vi "Bildaufnahme_Oben.vi"(8 "Fehler in":errorcluster, 11 "Cluster in":T1={"Initialisierung"={"Online?"=FALSE, "Grundpfad"=path "", "Kamera Oben"="", "IP-Adresse Flüssiglinse"="", "Flüssiglinse"=refnum, "Kamera Unten"="", "IP-Adresse SPS"="", "SPS-Verbindung"={"TCP Connection Ref"=refnum, "IP address"="", "timeout ms"=5000, "Connected?"=FALSE, "PLC Type"=enum."S7 1200", "Rack S7 400"=0, "Slot S7 400"=0, "PDU Size"=0, "connection semaphore"=refnum}, "IP-Adresse Lichtgitter"="", "Lichtgitter"=refnum, "Skalierungsfaktor"=0.0, "Bilder Oben"=[], "Bild Unten"=refnum, "Bild Ausschnitt Unten"=refnum}, "Einstellungen"={"Gesamtablauf gestartet"=FALSE, "i. O. Bilder speichern"=FALSE, "Bildspeicherung Offline"=FALSE, "Ausgewähltes Offline-Datum"="", "Ausgewähltes Offline-Teil"="", "Speicherpfad Bilder"=path ""}, "Artikeldaten"={"Artikelnummer"="", "Fertigungsauftrag"="", "Muster ISO"=refnum, "Belichtungszeit Referenzmarken"=0.0, "Fokus Referenzmarken"=0.0, "Belichtungszeit ISO"=0.0, "Fokus ISO"=0.0, "Belichtungszeit Unten"=0.0, "Kontaktanzahl"=0, "Aktueller Kontakt"=0, "Kontaktposition"={"x"=0.0, "y"=0.0}, "ISO-Muster nicht vorhanden"=FALSE, "Winkel ISO"=0.0, "Mittelpunkt ISO"={"x"=0.0, "y"=0.0}}, "Werte Kamera Oben"={"Koordinatensystem"={"Punkt x-Achse"={"X"=0.0, "Y"=0.0}, "Ursprung"={"X"=0.0, "Y"=0.0}, "Punkt y-Achse"={"X"=0.0, "Y"=0.0}}, "Position Kontakt"={"x"=0.0, "y"=0.0}, "Durchmesser Loch"=0.0, "Winkel Kontakt"=0.0, "Position Kontakt umgerechnet"={"x"=0.0, "y"=0.0}}, "Werte Kamera Unten"={"Prüfung Unten n. i. O."=FALSE}, "Werte Lichtgitter"={"Messwerte Referenzmarken"=[], "Mittelpunkt Referenzmarken"={"x"=0.0, "y"=0.0}, "Messwerte Kontakt"=[], "Offset"={"x"=0.0, "y"=0.0}}, "Rückmeldungen"={"Koordinaten ermittelt"=FALSE, "Vermessung Lichtgitter fertig"=FALSE, "Nachkontrolle Kamera Unten fertig"=FALSE}, "Fehler"={"Referenzen nicht gefunden"=FALSE, "Kontakt nicht gefunden"=FALSE, "Referenzen nicht in Lichtgitter"=FALSE, "Kontakt zu groß"=FALSE, "Kontakt zu klein"=FALSE}, "Statistik"={"Statistiken"=[]}, "Timer"={"Timer Start Position"=0, "Timer Start Lichtgitter"=0, "Timer Start Kamera Unten"=0}}) -> (0 "Fehler out":errorcluster, 3 "Cluster out":T1={"Initialisierung"={"Online?"=FALSE, "Grundpfad"=path "", "Kamera Oben"="", "IP-Adresse Flüssiglinse"="", "Flüssiglinse"=refnum, "Kamera Unten"="", "IP-Adresse SPS"="", "SPS-Verbindung"={"TCP Connection Ref"=refnum, "IP address"="", "timeout ms"=5000, "Connected?"=FALSE, "PLC Type"=enum."S7 1200", "Rack S7 400"=0, "Slot S7 400"=0, "PDU Size"=0, "connection semaphore"=refnum}, "IP-Adresse Lichtgitter"="", "Lichtgitter"=refnum, "Skalierungsfaktor"=0.0, "Bilder Oben"=[], "Bild Unten"=refnum, "Bild Ausschnitt Unten"=refnum}, "Einstellungen"={"Gesamtablauf gestartet"=FALSE, "i. O. Bilder speichern"=FALSE, "Bildspeicherung Offline"=FALSE, "Ausgewähltes Offline-Datum"="", "Ausgewähltes Offline-Teil"="", "Speicherpfad Bilder"=path ""}, "Artikeldaten"={"Artikelnummer"="", "Fertigungsauftrag"="", "Muster ISO"=refnum, "Belichtungszeit Referenzmarken"=0.0, "Fokus Referenzmarken"=0.0, "Belichtungszeit ISO"=0.0, "Fokus ISO"=0.0, "Belichtungszeit Unten"=0.0, "Kontaktanzahl"=0, "Aktueller Kontakt"=0, "Kontaktposition"={"x"=0.0, "y"=0.0}, "ISO-Muster nicht vorhanden"=FALSE, "Winkel ISO"=0.0, "Mittelpunkt ISO"={"x"=0.0, "y"=0.0}}, "Werte Kamera Oben"={"Koordinatensystem"={"Punkt x-Achse"={"X"=0.0, "Y"=0.0}, "Ursprung"={"X"=0.0, "Y"=0.0}, "Punkt y-Achse"={"X"=0.0, "Y"=0.0}}, "Position Kontakt"={"x"=0.0, "y"=0.0}, "Durchmesser Loch"=0.0, "Winkel Kontakt"=0.0, "Position Kontakt umgerechnet"={"x"=0.0, "y"=0.0}}, "Werte Kamera Unten"={"Prüfung Unten n. i. O."=FALSE}, "Werte Lichtgitter"={"Messwerte Referenzmarken"=[], "Mittelpunkt Referenzmarken"={"x"=0.0, "y"=0.0}, "Messwerte Kontakt"=[], "Offset"={"x"=0.0, "y"=0.0}}, "Rückmeldungen"={"Koordinaten ermittelt"=FALSE, "Vermessung Lichtgitter fertig"=FALSE, "Nachkontrolle Kamera Unten fertig"=FALSE}, "Fehler"={"Referenzen nicht gefunden"=FALSE, "Kontakt nicht gefunden"=FALSE, "Referenzen nicht in Lichtgitter"=FALSE, "Kontakt zu groß"=FALSE, "Kontakt zu klein"=FALSE}, "Statistik"={"Statistiken"=[]}, "Timer"={"Timer Start Position"=0, "Timer Start Lichtgitter"=0, "Timer Start Kamera Unten"=0}})   [LabVIEW 2024]
doc: "Nimmt die Bilder für die Prüfung Oben auf, bzw. lädt die Bilder aus den Dateien wenn im \"Offline-Modus\"."
uses:
  Typdefinitionen/Cluster.ctl
  <vilib>/userDefined/High Color/IMAQdx.ctl
  <vilib>/DATA AHEAD/SP7/typedefs/S7 Connection.ctl
  <vilib>/DATA AHEAD/SP7/typedefs/PLC Type.ctl
  <vilib>/vision/Image Controls.llb/IMAQ Image.ctl
  Typdefinitionen/Koordinatensystem.ctl
  Typdefinitionen/Statistik.ctl
  <vilib>/vision/driver/IMAQdx.llb/IMAQdx Buffer Number Mode.ctl
  <resource>/objmgr/imaqdx.rc
  <vilib>/vision/driver/NI_Vision_Acquisition_Software.lvlib
  <vilib>/vision/NI_Vision_Development_Module.lvlib
  <vilib>/DATA AHEAD/SP7/SP7.lvlib
panel:
  in  "Zeit für Fokus":u32=300
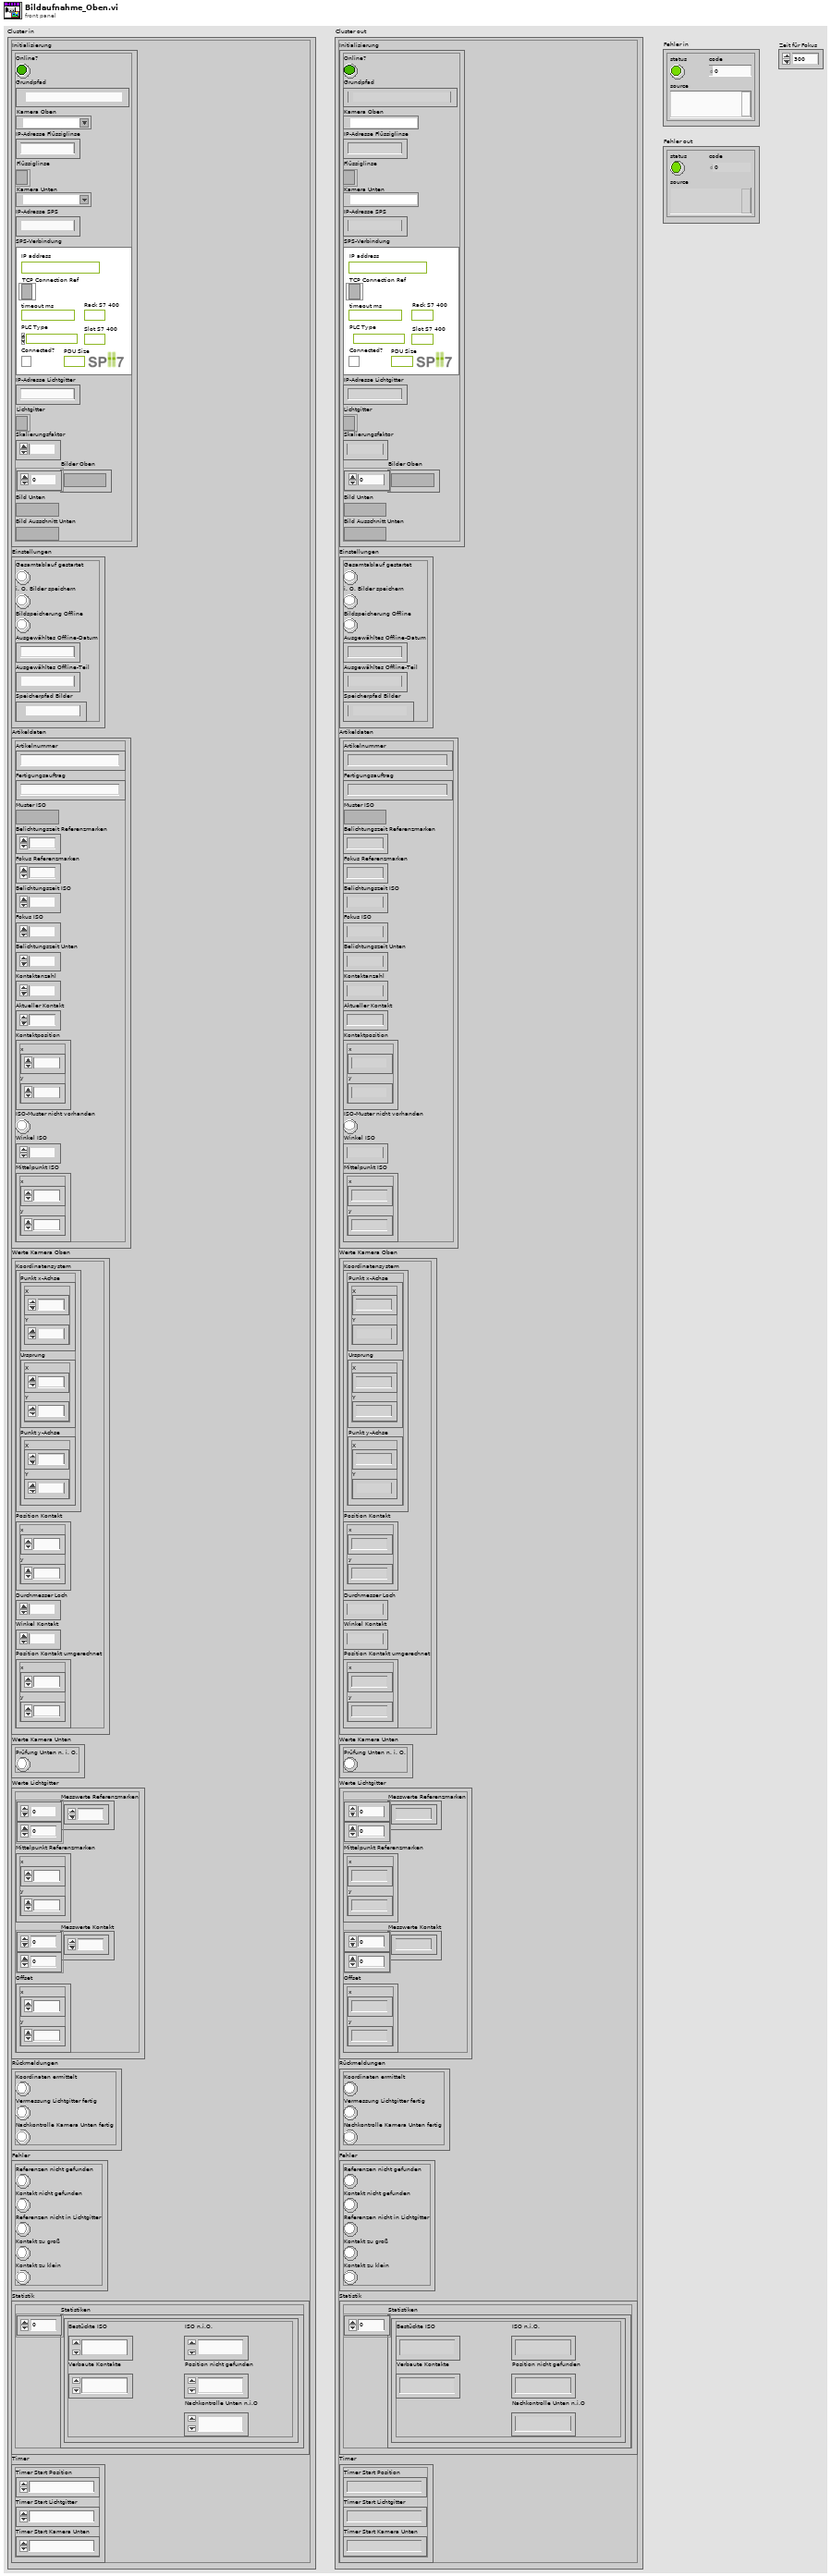
[diagram p1: front panel]
types:
  T1 = typedef "Cluster.ctl" = cluster{"Initialisierung":cluster{"Online?":bool, "Grundpfad":path, "Kamera Oben":T2, "IP-Adresse Flüssiglinse":string, "Flüssiglinse":refnum<k5>, "Kamera Unten":T2, "IP-Adresse SPS":string, "SPS-Verbindung":T3, "IP-Adresse Lichtgitter":string, "Lichtgitter":refnum<k5>, "Skalierungsfaktor":dbl, "Bilder Oben":T6[], "Bild Unten":T6, "Bild Ausschnitt Unten":T6}, "Einstellungen":cluster{"Gesamtablauf gestartet":bool, "i. O. Bilder speichern":bool, "Bildspeicherung Offline":bool, "Ausgewähltes Offline-Datum":string, "Ausgewähltes Offline-Teil":string, "Speicherpfad Bilder":path}, "Artikeldaten":cluster{"Artikelnummer":string, "Fertigungsauftrag":string, "Muster ISO":T6, "Belichtungszeit Referenzmarken":dbl, "Fokus Referenzmarken":dbl, "Belichtungszeit ISO":dbl, "Fokus ISO":dbl, "Belichtungszeit Unten":dbl, "Kontaktanzahl":u32, "Aktueller Kontakt":i16, "Kontaktposition":cluster{"x":sgl, "y":sgl}, "ISO-Muster nicht vorhanden":bool, "Winkel ISO":sgl, "Mittelpunkt ISO":cluster{"x":dbl, "y":dbl}}, "Werte Kamera Oben":cluster{"Koordinatensystem":T7, "Position Kontakt":cluster{"x":dbl, "y":dbl}, "Durchmesser Loch":dbl, "Winkel Kontakt":dbl, "Position Kontakt umgerechnet":cluster{"x":dbl, "y":dbl}}, "Werte Kamera Unten":cluster{"Prüfung Unten n. i. O.":bool}, "Werte Lichtgitter":cluster{"Messwerte Referenzmarken":dbl[][], "Mittelpunkt Referenzmarken":cluster{"x":dbl, "y":dbl}, "Messwerte Kontakt":dbl[][], "Offset":cluster{"x":dbl, "y":dbl}}, "Rückmeldungen":cluster{"Koordinaten ermittelt":bool, "Vermessung Lichtgitter fertig":bool, "Nachkontrolle Kamera Unten fertig":bool}, "Fehler":cluster{"Referenzen nicht gefunden":bool, "Kontakt nicht gefunden":bool, "Referenzen nicht in Lichtgitter":bool, "Kontakt zu groß":bool, "Kontakt zu klein":bool}, "Statistik":cluster{"Statistiken":T8[]}, "Timer":cluster{"Timer Start Position":u32, "Timer Start Lichtgitter":u32, "Timer Start Kamera Unten":u32}}
  T2 = typedef "IMAQdx.ctl" = refnum<k21>
  T3 = typedef "SP7.lvlib/S7 Connection.ctl" = cluster{"TCP Connection Ref":refnum<k5>, "IP address":string, "timeout ms":i32, "Connected?":bool, "PLC Type":T4, "Rack S7 400":u8, "Slot S7 400":u8, "PDU Size":u16, "connection semaphore":T5}
  T4 = typedef "SP7.lvlib/PLC Type.ctl" = enum16{"S7 200", "S7 300/400", "S7 1200", "S7 1500", "LOGO!8"}
  T5 = typedef "Semaphore RefNum" = refnum<k1>
  T6 = typedef "IMAQ Image.ctl" = refnum<image>
  T7 = typedef "Koordinatensystem.ctl" = cluster{"Punkt x-Achse":cluster{"X":sgl, "Y":sgl}, "Ursprung":cluster{"X":sgl, "Y":sgl}, "Punkt y-Achse":cluster{"X":sgl, "Y":sgl}}
  T8 = typedef "Statistik.ctl" = cluster{"Bestückte ISO":u32, "Verbaute Kontakte":u32, "ISO n.i.O.":u32, "Nachkontrolle Unten n.i.O":u32, "Position nicht gefunden":u32}
  T9 = typedef "IMAQ Rectangle" = cluster{"Left":i32, "Top":i32, "Right":i32, "Bottom":i32, "Rotation":dbl}
  T10 = typedef "NI_Vision_Acquisition_Software.lvlib/IMAQdx Buffer Number Mode.ctl" = enum32{"Next", "Last", "Buffer Number", "Every", "Last New"}
  T11 = typedef "ROI Descriptor" = cluster{"Global Rectangle":i32[], "Contours":cluster{"ID":enum32{"External", "Internal"}, "Type":u32, "Coordinates":i32[]}[]}
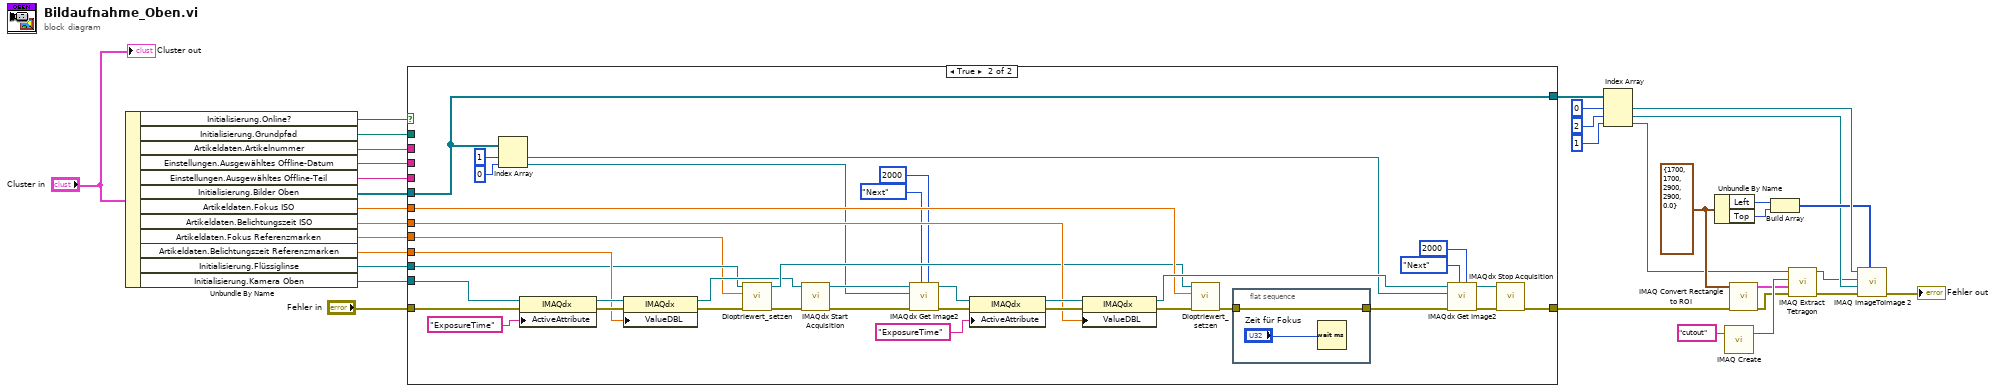
[diagram p0: block diagram]
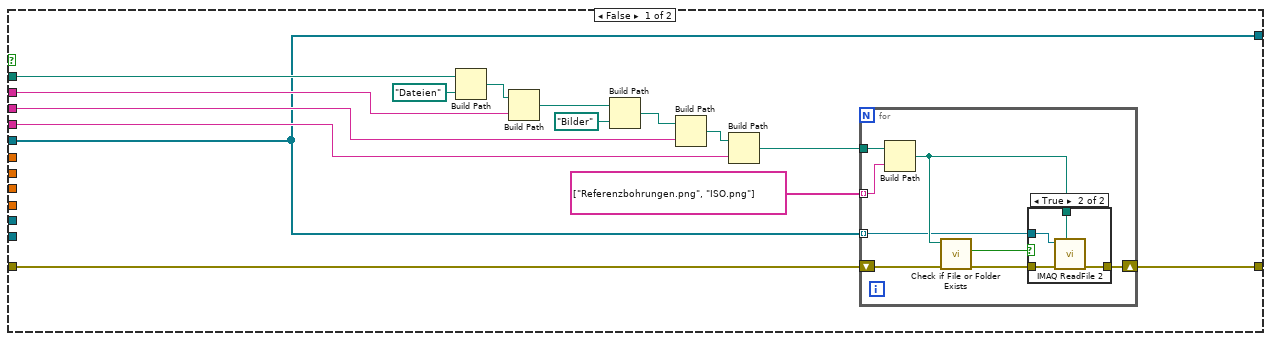
[diagram p2: hidden frame]
diagram:
  w9 = T9 {"Left"=1700, "Top"=1700, "Right"=2900, "Bottom"=2900, "Rotation"=0.0} ("Rectangle")
  n1 = Unbundle By Name("Cluster in") -> ("Initialisierung.Online?"=w4:bool, "Initialisierung.Grundpfad"=w33:path, "Artikeldaten.Artikelnummer"=w32:string, "Einstellungen.Ausgewähltes Offline-Datum"=w30:string, "Einstellungen.Ausgewähltes Offline-Teil"=w31:string, "Initialisierung.Bilder Oben"=w29:T6[], "Artikeldaten.Fokus ISO"=w21:dbl, "Artikeldaten.Belichtungszeit ISO"=w23:dbl, "Artikeldaten.Fokus Referenzmarken"=w1:dbl, "Artikeldaten.Belichtungszeit Referenzmarken"=w22:dbl, "Initialisierung.Flüssiglinse"=w2:refnum<k5>, "Initialisierung.Kamera Oben"=w3:T2)
  n2 = case shown="True" w4 {
    tunnel: w33 -> [w40 _]
    tunnel: w32 -> [w37 _]
    tunnel: w30 -> [w45 _]
    tunnel: w31 -> [w46 _]
    tunnel: w29 -> [w34 w66]
    tunnel: "Fehler in" -> [w42 w82]
    tunnel: [w35 w96] -> w26
    tunnel: [w34 w66] -> w24
    tunnel: w23 -> [_ w79]
    tunnel: w22 -> [_ w80]
    tunnel: w21 -> [_ w78]
    tunnel: w3 -> [_ w64]
    tunnel: w2 -> [_ w63]
    tunnel: w1 -> [_ w62]
    frame False {
      n3 = Build Path(base path=w40, name or relative path=path "Dateien") -> (appended path=w39:path)
      n4 = Build Path(base path=w39, name or relative path=w37) -> (appended path=w48:path)
      n5 = Build Path(base path=w48, name or relative path=path "Bilder") -> (appended path=w41:path)
      n6 = Build Path(base path=w41, name or relative path=w45) -> (appended path=w47:path)
      n7 = Build Path(base path=w47, name or relative path=w46) -> (appended path=w44:path)
      n8 = for {
        tunnel: w34 -> [w50] mode=indexing
        shift-right: [w54] -> w35
        shift-left: w42 -> [w53]
        tunnel: w44 -> [w56]
        tunnel: string[] ["Referenzbohrungen.png", "ISO.png"] -> [w55] mode=indexing
        n9 = Build Path(base path=w56, name or relative path=w55) -> (appended path=w51:path)
        n10 = call <vilib>:"Check if File or Folder Exists.vi"("error in (no error)"=w53, "path"=w51) -> ("error out"=w52:errorcluster, "file or folder exists?"=w49:bool)  [unwired: 7 in, 1 out]
        n11 = case shown="True" w49 {
          tunnel: [w57 w61] -> w54
          tunnel: w52 -> [w57 w60]
          tunnel: w51 -> [_ w59]
          tunnel: w50 -> [_ w58]
          frame False {
          }
          frame True {
            n12 = call "IMAQ ReadFile 2"("File Path"=w59, "error in (no error)"=w60, "Image"=w58) -> ("error out"=w61:errorcluster)  [unwired: 4 in, 4 out]
          }
        }
      }
    }
    frame True {
      n13 = Index Array(array=w66, index #1=1 ("index"), index #2=0 ("index")) -> (element #1=w67:T6, element #2=w68:T6)
      n14 = property class="IMAQdx"(reference=w64, error in=w82, "ActiveAttribute"="ExposureTime") -> (reference out=w85:T2, error out=w84:errorcluster)
      n15 = property class="IMAQdx"(reference=w85, error in=w84, "ValueDBL"=w80) -> (reference out=w65:T2, error out=w86:errorcluster)
      n16 = call "Dioptriewert_setzen.vi"("Fehler in"=w86, "Dioptrie-Wert"=w62, "Flüssiglinse in"=w63) -> ("Fehler out"=w83:errorcluster, "Flüssiglinse out"=w77:refnum<k5>)  [unwired: 7 in]
      n17 = call <vilib>:"IMAQdx Start Acquisition.vi"("error in"=w83, "Session In"=w65) -> ("error out"=w74:errorcluster, "Session Out"=w72:T2)  [unwired: 8 in]
      n18 = call <vilib>:"IMAQdx Get Image2.vi"("Timeout (ms)"=2000, "Buffer Number Mode (Next)"=IMAQdx_Buffer_Number_Mode."Next", "error in"=w74, "Image In"=w68, "Session In"=w72) -> ("error out"=w73:errorcluster, "Session Out"=w71:T2)  [unwired: 3 in, 2 out]
      n19 = property class="IMAQdx"(reference=w71, error in=w73, "ActiveAttribute"="ExposureTime") -> (reference out=w94:T2, error out=w95:errorcluster)
      n20 = property class="IMAQdx"(reference=w94, error in=w95, "ValueDBL"=w79) -> (reference out=w89:T2, error out=w92:errorcluster)
      n21 = call "Dioptriewert_setzen.vi"("Fehler in"=w92, "Dioptrie-Wert"=w78, "Flüssiglinse in"=w77) -> ("Fehler out"=w91:errorcluster)  [unwired: 7 in, 1 out]
      n22 = flat-sequence {
        tunnel: w91 -> [w100]
        tunnel: [w100] -> w90
        frame #0 {
          n23 = Wait (ms)(milliseconds to wait="Zeit für Fokus") -> ()  [unwired: 1 out]
        }
      }
      n24 = call <vilib>:"IMAQdx Get Image2.vi"("Timeout (ms)"=2000, "Buffer Number Mode (Next)"=IMAQdx_Buffer_Number_Mode."Next", "error in"=w90, "Image In"=w67, "Session In"=w89) -> ("error out"=w98:errorcluster, "Session Out"=w97:T2)  [unwired: 3 in, 2 out]
      n25 = call <vilib>:"IMAQdx Stop Acquisition.vi"("error in"=w98, "Session In"=w97) -> ("error out"=w96:errorcluster)  [unwired: 8 in, 1 out]
    }
  }
  n26 = Index Array(array=w24, index #1=0 ("index"), index #2=2 ("index"), index #3=1 ("index")) -> (element #1=w19:T6, element #2=w8:T6, element #3=w7:T6)
  n27 = Unbundle By Name(w9) -> ("Left"=w16:i32, "Top"=w15:i32)
  n28 = call "IMAQ Create"("Image Name"="cutout") -> ("New Image"=w20:T6)  [unwired: 4 in, 1 out]
  n29 = call "IMAQ Convert Rectangle to ROI"("error in (no error)"=w26, "Rectangle"=w9) -> ("error out"=w17:errorcluster, "ROI Descriptor"=w18:T11)  [unwired: 7 in]
  n30 = Build Array(w16, w15) -> (w14:i32[])
  n31 = call-poly "IMAQ Extract Tetragon"("error in (no error)"=w17, "ROI Descriptor"=w18, "Image Dst"=w20, "Image Src"=w7) -> ("error out"=w5:errorcluster, "Image Dst Out"=w6:T6)  [unwired: 6 in]
  n32 = call "IMAQ ImageToImage 2"("Offset Left/Top"=w14, "error in (no error)"=w5, "Image Dst"=w8, "Image Src (Small)"=w6, "Image Src (Large)"=w19) -> ("error out"=→"Fehler out":errorcluster)  [unwired: 5 in, 1 out]
  "Cluster out" <- "Cluster in"
